vi "Ethernet IP Custom Device Main Page.vi"(8 "error in (no error)":errorcluster, 11 "Node Ptr":T1 format="%.0x") -> (0 "error out":errorcluster)   [LabVIEW 2011, in "Ethernet IP Custom Device Custom Device.lvlib"]
uses:
  Ethernet IP Custom Device Custom Device.lvlib
  <vilib>/NI Veristand/Custom Device API/Custom Device Item Ref.ctl
  <vilib>/NI Veristand/Custom Device API/Custom Device Channel.ctl
  <vilib>/NI Veristand/Custom Device API/Custom Device Channel Type.ctl
  Ethernet IP Global Strings.vi
  <vilib>/NI Veristand/Custom Device API/Get Item Property (I32).vi
  <vilib>/NI Veristand/Custom Device API/Set Item Property (String).vi
  <vilib>/NI Veristand/Custom Device API/Set Item Property (Path).vi
  Ethernet IP Global GUIDs.vi
  <vilib>/NI Veristand/Custom Device API/Set Item Property (I32).vi
  <vilib>/NI Veristand/Custom Device API/Get Item Property (String).vi
  <vilib>/NI Veristand/Custom Device API/Get Item Property (Path).vi
  <vilib>/NI Veristand/Custom Device API/Custom Device API.lvlib
panel:
  in  "Import Selected File":bool
  in  "Path to L5K file":path
  in  "Update Rate (ms)":i32
  in  "Communication Timeout (ms)":i32
  in  "Logix Slot":u16
  in  "Backplane Port":u16
  in  "PLC Address (IP Address)":string
  in  "Header":cluster{"Section Name":string}={"Section Name"="Custom Device Item Settings"}
  in  "Description":string
  in  "Name":string
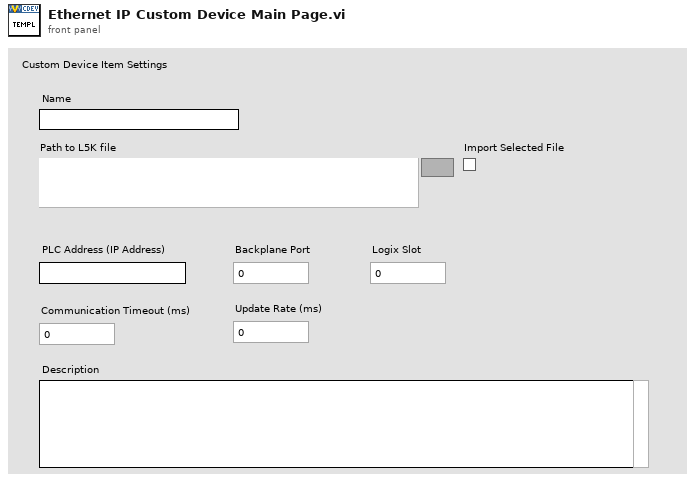
[diagram p1: front panel]
types:
  T1 = typedef "Custom Device API.lvlib/Custom Device Item Ref.ctl" = u64
  T2 = enum8{"Enabled", "Disabled", "Disabled and Grayed Out"}
  T3 = typedef "Custom Device API.lvlib/Custom Device Item Info.ctl" = cluster{"Name":string, "Is Channel":bool, "GUID":string}
  T4 = typedef "Custom Device API.lvlib/Custom Device Channel.ctl" = cluster{"Type":T5, "Units":string, "Default Value":dbl, "Faultable":bool, "Scalable":bool}
  T5 = typedef "Custom Device API.lvlib/Custom Device Channel Type.ctl" = enum16{"Input", "Output"}
  T6 = typedef "Custom Device API.lvlib/Custom Device Commands.ctl" = enum16{"Default", "Item renamed", "Shutdown", "Dynamic button pressed"}
  T7 = typedef "Ethernet IP Custom Device Custom Device.lvlib/L5K Internal Data.ctl" = cluster{"L5K Entire String":string, "L5K Extractred String Array":string[], "IP address from CommPath":string, "Configured Tags":T8[], "Data String Array":string[], "Unconfigured Tags":T8[], "# Tags":i32}
  T8 = typedef "Ethernet IP Custom Device Custom Device.lvlib/L5K Tag.ctl" = cluster{"Tag Name":string, "Data Type":T9, "Data Type String":string, "Array Size":i32, "Description":string, "Input?":bool, "Channel Name":string}
  T9 = typedef "Ethernet IP Custom Device Custom Device.lvlib/L5K Data Types.ctl" = enum16{"SINT", "INT", "DINT", "REAL", "BOOL"}
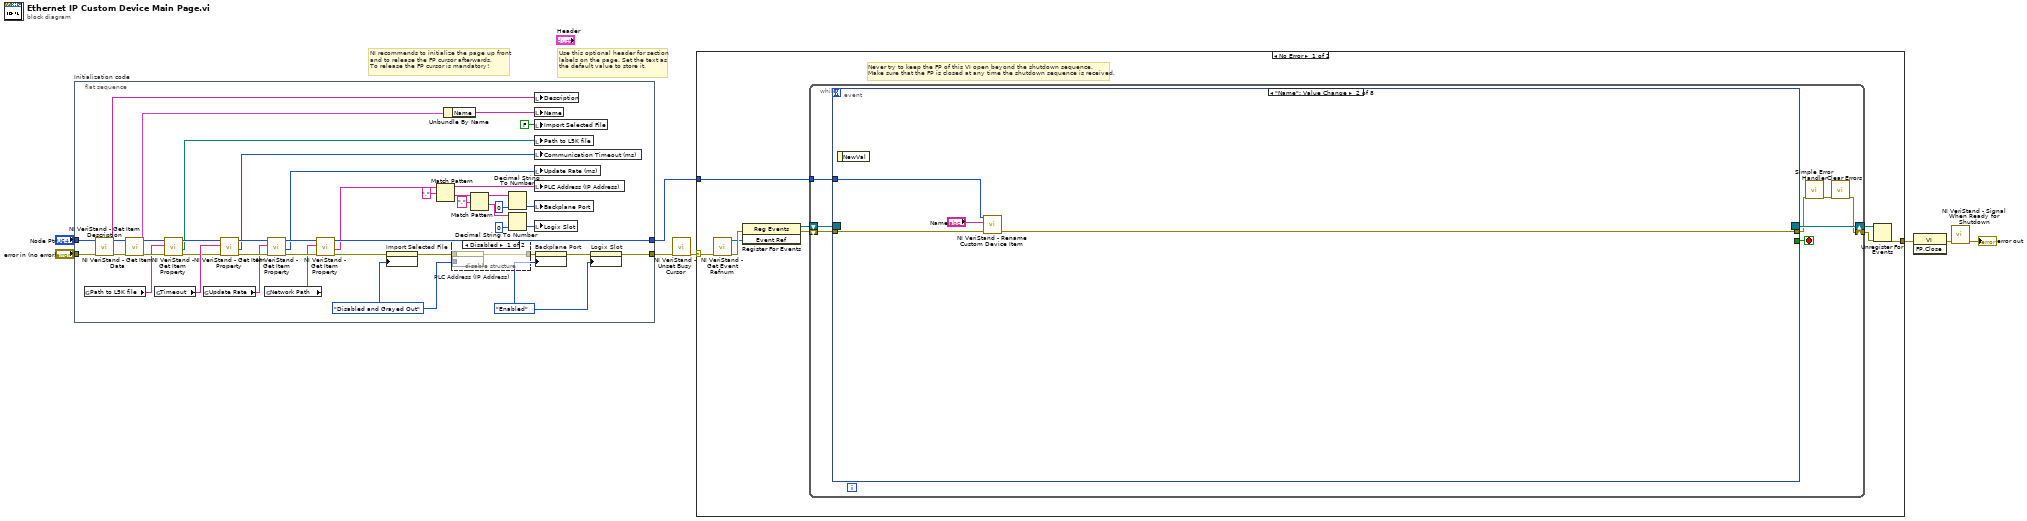
[diagram p0: block diagram]
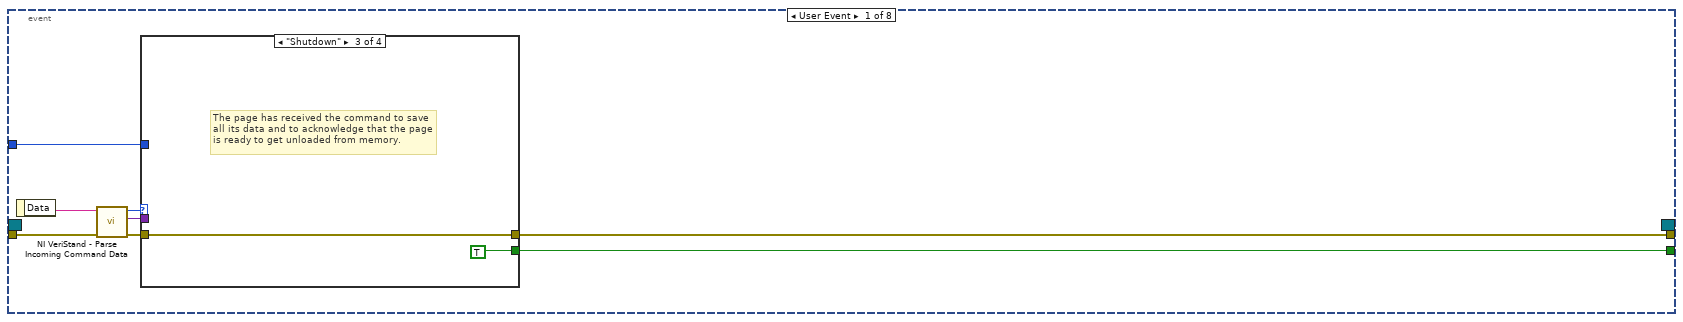
[diagram p2: hidden frame]
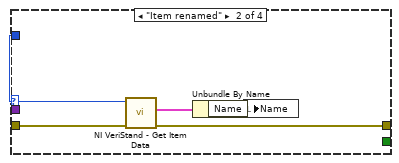
[diagram p4: hidden frame]
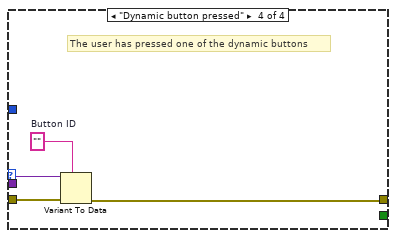
[diagram p5: hidden frame]
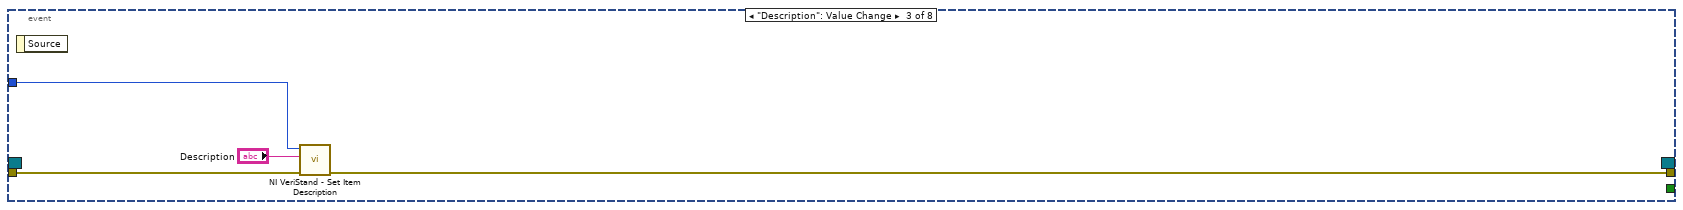
[diagram p6: hidden frame]
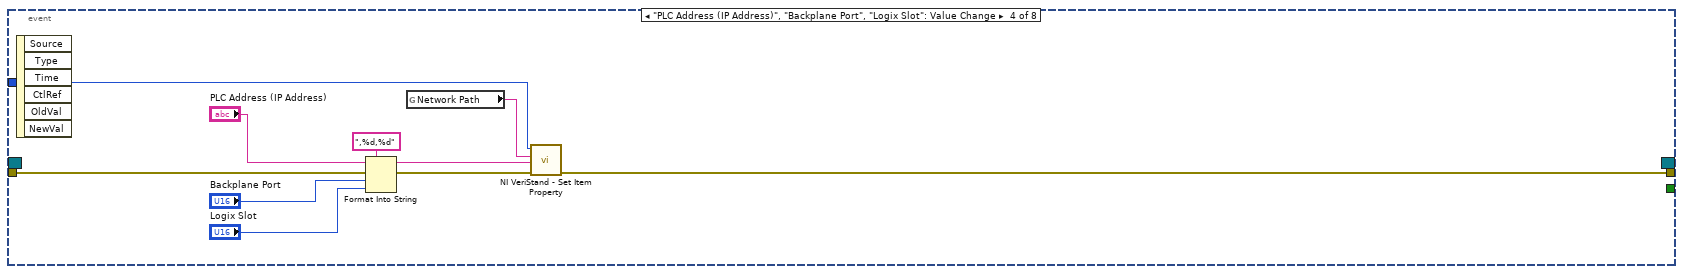
[diagram p7: hidden frame]
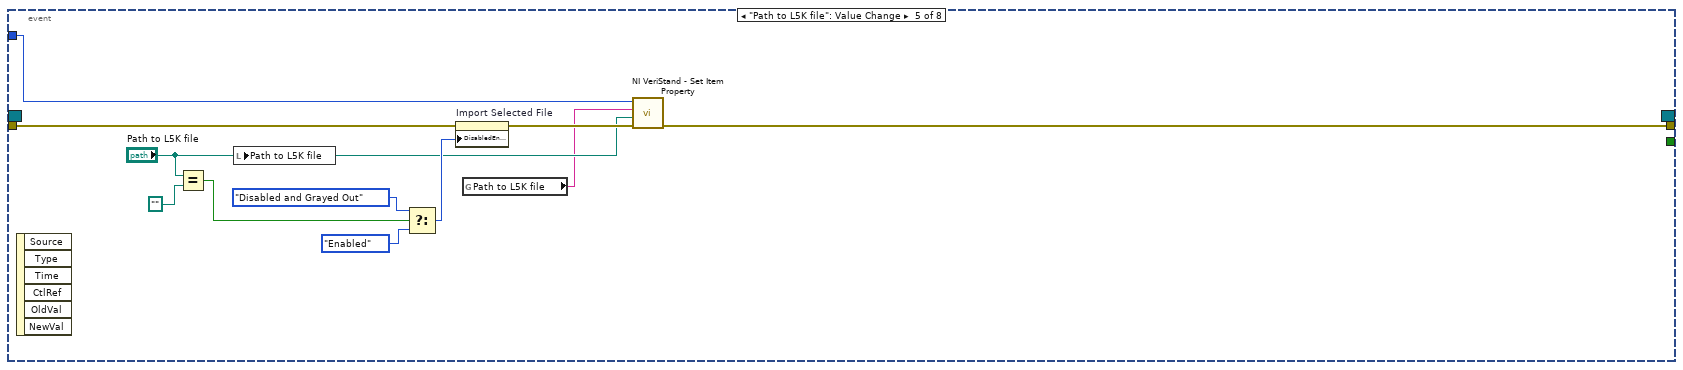
[diagram p8: hidden frame]
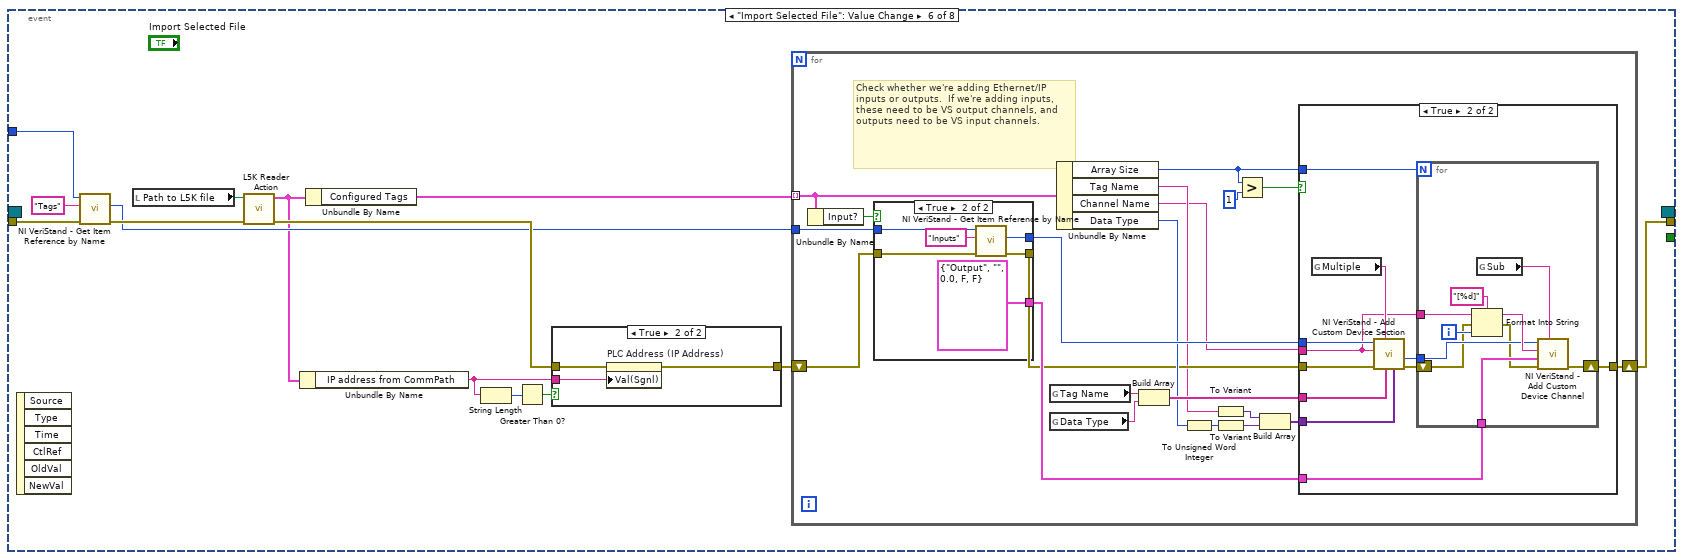
[diagram p9: hidden frame]
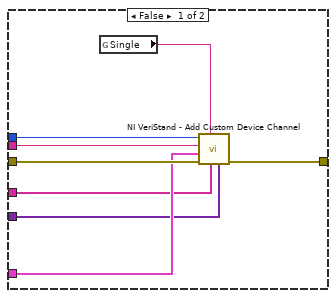
[diagram p10: hidden frame]
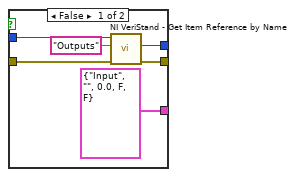
[diagram p11: hidden frame]
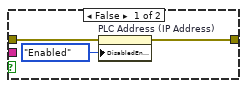
[diagram p12: hidden frame]
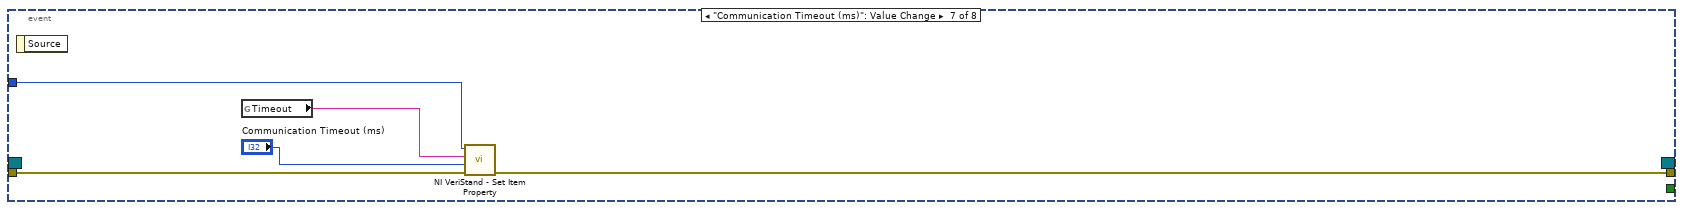
[diagram p13: hidden frame]
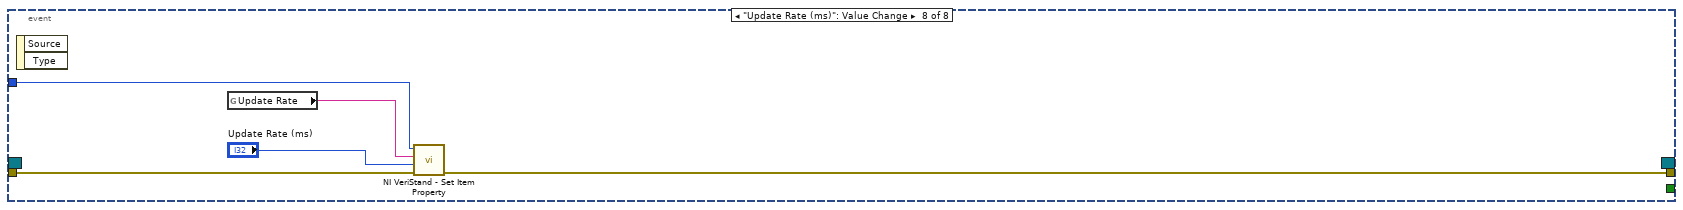
[diagram p14: hidden frame]
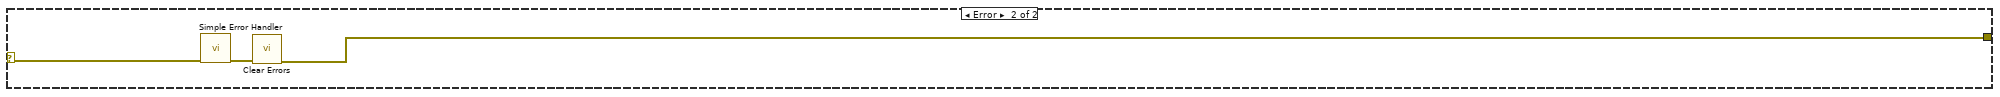
[diagram p15: hidden frame]
diagram:
  # "Use this optional header for section labels on the page. Set the text as the default value to store it."
  # "NI recommends to initialize the page up front\nand to release the FP cursor afterwards.\nTo release the FP cursor is mandatory!"
  n1 = flat-sequence "Initialization code" {
    tunnel: "error in (no error)" -> [w49]
    tunnel: "Node Ptr" -> [w48]
    tunnel: [w20] -> w4
    tunnel: [w27] -> w1
    frame #0 {
      w19 = T2."Enabled" ("Disabled")
      w16 = T2."Disabled and Grayed Out" ("Disabled")
      n2 = global read "Ethernet IP Global Strings.vi" "Path to L5K file"() -> (w10:string)
      n3 = call <vilib>:"NI VeriStand - Get Item Description.vi"("error in (no error)"=w49, "Item Ref in"=w48) -> ("error out"=w46:errorcluster, "Description"=w47:string, "Item Ref out"=w50:T1)  [unwired: 7 out]
      n4 = call <vilib>:"NI VeriStand - Get Item Data.vi"("error in (no error)"=w46, "Item Ref in"=w50) -> ("error out"=w13:errorcluster, "Item Info"=w45:T3, "Item Ref out"=w15:T1)  [unwired: 7 out]
      n5 = global read "Ethernet IP Global Strings.vi" "Timeout"() -> (w33:string)
      n6 = call-poly <vilib>:"NI VeriStand - Get Item Property.vi"("error in (no error)"=w13, "Property Name"=w10, "Item Ref in"=w15) -> ("error out"=w12:errorcluster, "Value"=w9:path, "Item Ref out"=w14:T1)  [unwired: 5 in, 1 out]
      n7 = global read "Ethernet IP Global Strings.vi" "Update Rate"() -> (w32:string)
      n8 = call-poly <vilib>:"NI VeriStand - Get Item Property.vi"("error in (no error)"=w12, "Property Name"=w33, "Item Ref in"=w14) -> ("error out"=w41:errorcluster, "Value"=w30:i32, "Item Ref out"=w43:T1)  [unwired: 5 in, 1 out]
      n9 = global read "Ethernet IP Global Strings.vi" "Network Path"() -> (w31:string)
      n10 = call-poly <vilib>:"NI VeriStand - Get Item Property.vi"("error in (no error)"=w41, "Property Name"=w32, "Item Ref in"=w43) -> ("error out"=w40:errorcluster, "Value"=w28:i32, "Item Ref out"=w42:T1)  [unwired: 5 in, 1 out]
      n11 = call-poly <vilib>:"NI VeriStand - Get Item Property.vi"("error in (no error)"=w40, "Property Name"=w31, "Item Ref in"=w42) -> ("error out"=w18:errorcluster, "Value"=w24:string, "Item Ref out"=w27:T1)  [unwired: 5 in, 1 out]
      n12 = property on="Import Selected File" class="Bool (strict)"(error in=w18, "DisabledEnum"=w16) -> (error out=w17:errorcluster)  [unwired: 1 in, 1 out]
      n13 = Match Pattern(string=w24, regular expression=",") -> (before substring=w25:string, after substring=w23:string)  [unwired: 1 in, 2 out]
      n14 = Unbundle By Name(w45) -> ("Name"=w44:string)
      n15 = disable-structure shown="Disabled" {
        disable-tunnel: [w53 w54] -> w22
        disable-tunnel: w17 -> [w52 w54]
        disable-tunnel: w16 -> [w51 _]
        frame Disabled {
          n16 = property on="PLC Address (IP Address)" class="Str"(error in=w52, "DisabledEnum"=w51) -> (error out=w53:errorcluster)  [unwired: 1 in, 1 out]
        }
        frame Enabled {
        }
      }
      n17 = Match Pattern(string=w23, regular expression=",") -> (before substring=w37:string, after substring=w36:string)  [unwired: 1 in, 2 out]
      n18 = Decimal String To Number(string=w37, default (0L)=u16 0 ("default (0 I32)")) -> (number=w34:u16)  [unwired: 1 in, 1 out]
      n19 = Decimal String To Number(string=w36, default (0L)=u16 0 ("default (0 I32)")) -> (number=w29:u16)  [unwired: 1 in, 1 out]
      n20 = local write "Description"(w47) -> ()
      n21 = local write "Name"(w44) -> ()
      n22 = local write "Import Selected File"(FALSE ("Import Selected File")) -> ()
      n23 = local write "Path to L5K file"(w9) -> ()
      n24 = local write "Communication Timeout (ms)"(w30) -> ()
      n25 = local write "Update Rate (ms)"(w28) -> ()
      n26 = local write "PLC Address (IP Address)"(w25) -> ()
      n27 = local write "Backplane Port"(w34) -> ()
      n28 = local write "Logix Slot"(w29) -> ()
      n29 = property on="Backplane Port" class="DigNum (strict)"(error in=w22, "DisabledEnum"=w19) -> (error out=w21:errorcluster)  [unwired: 1 in, 1 out]
      n30 = property on="Logix Slot" class="DigNum (strict)"(error in=w21, "DisabledEnum"=w19) -> (error out=w20:errorcluster)  [unwired: 1 in, 1 out]
    }
  }
  n31 = call <vilib>:"NI VeriStand - Unset Busy Cursor.vi"("error in (no error)"=w4) -> ("error out"=w3:errorcluster)  [unwired: 10 out]
  n32 = case shown="No Error" w3 {
    selector: w3 -> [w55 w215]
    tunnel: [w60 w213] -> w8
    tunnel: w1 -> [w56 _]
    frame No Error {
      # "Never try to keep the FP of this VI open beyond the shutdown sequence.\nMake sure that the FP is closed at any time the shutdown sequence is received."
      n33 = call <vilib>:"NI VeriStand - Get Event Refnum.vi"("error in (no error)"=w55) -> ("error out"=w63:errorcluster, "Event Ref"=w59:refnum<user-event>)  [unwired: 9 out]
      n34 = register-events(error in=w63, w59) -> (reference out=w57:refnum<event-registration>, error out=w58:errorcluster)  [unwired: 1 in]
      n35 = while {
        tunnel: w56 -> [w67]
        shift-right: [w64] -> w61
        shift-left: w58 -> [w70]
        shift-right: [w71] -> w62
        shift-left: w57 -> [w69]
        stop <- w68 stop-if-true
        n36 = event shown="[1] \"Name\": Value Change" {
          selector: w69 -> [_ _ _ _ _ _ _ _]
          dyn-events: [_ _ _ _ _ _ _ _] -> w71
          timeout: _ -> [_ _ _ _ _ _ _ _]
          tunnel: w70 -> [w79 w95 w98 w105 w115 w126 w204 w210]
          tunnel: [w75 _ _ _ _ _ _ _] -> w68
          tunnel: [w74 w94 w97 w109 w113 w128 w207 w212] -> w66
          tunnel: w67 -> [w73 w93 w99 w108 w112 w127 w206 w211]
          event User Event {
            n37 = event-data() -> ("Data"=w78:string)  [unwired: 1 out]
            n38 = call <vilib>:"NI VeriStand - Parse Incoming Command Data.vi"("error in (no error)"=w79, "Incoming data"=w78) -> ("error out"=w77:errorcluster, "Outgoing data"=w72:variant, "Action"=w76:T6)  [unwired: 7 out]
            n39 = case shown="\"Shutdown\"" w76 {
              tunnel: w77 -> [w80 w85 w86 w91]
              tunnel: [_ _ TRUE _] -> w75
              tunnel: [w80 w82 w86 w88] -> w74
              tunnel: w73 -> [_ w84 _ _]
              tunnel: w72 -> [_ _ _ w90]
              frame "Default", Default {
              }
              frame "Item renamed" {
                n40 = call <vilib>:"NI VeriStand - Get Item Data.vi"("error in (no error)"=w85, "Item Ref in"=w84) -> ("error out"=w82:errorcluster, "Item Info"=w83:T3)  [unwired: 8 out]
                n41 = Unbundle By Name(w83) -> ("Name"=w81:string)
                n42 = local write "Name"(w81) -> ()
              }
              frame "Shutdown" {
                # "The page has received the command to save all its data and to acknowledge that the page is ready to get unloaded from memory."
              }
              frame "Dynamic button pressed" {
                w89 = ""  # Button ID
                # "The user has pressed one of the dynamic buttons"
                n43 = Variant To Data(error in=w91, type=w89, Variant=w90) -> (error out=w88:errorcluster)  [unwired: 1 out]
              }
            }
          }
          event "Name": Value Change {
            n44 = event-data() -> ()  [unwired: 2 out]
            n45 = call <vilib>:"NI VeriStand - Rename Custom Device Item.vi"("error in (no error)"=w95, "New Name"="Name", "Item Ref in"=w93) -> ("error out"=w94:errorcluster)  [unwired: 8 out]
          }
          event "Description": Value Change {
            n46 = event-data() -> ()  [unwired: 2 out]
            n47 = call <vilib>:"NI VeriStand - Set Item Description.vi"("error in (no error)"=w98, "Description"="Description", "Item Ref in"=w99) -> ("error out"=w97:errorcluster)  [unwired: 8 out]
          }
          event "PLC Address (IP Address)", "Backplane Port", "Logix Slot": Value Change {
            n48 = event-data() -> ()  [unwired: 7 out]
            n49 = Format Into String(format string=",%d,%d", initial string="PLC Address (IP Address)", error in=w105, "Backplane Port", "Logix Slot") -> (resulting string=w103:string, error out=w104:errorcluster)
            n50 = global read "Ethernet IP Global Strings.vi" "Network Path"() -> (w107:string)
            n51 = call-poly <vilib>:"NI VeriStand - Set Item Property.vi"("error in (no error)"=w104, "Value"=w103, "Property Name"=w107, "Item Ref in"=w108) -> ("error out"=w109:errorcluster)  [unwired: 5 in, 2 out]
          }
          event "Path to L5K file": Value Change {
            n52 = event-data() -> ()  [unwired: 7 out]
            n53 = Equal?(x="Path to L5K file", y=path "") -> (x = y?=w119:bool)
            n54 = local write "Path to L5K file"("Path to L5K file") -> ()
            n55 = Select(t=T2."Disabled and Grayed Out" ("Disabled"), s=w119, f=T2."Enabled" ("Disabled")) -> (s? t:f=w116:T2)
            n56 = property on="Import Selected File" class="Bool (strict)"(error in=w115, "DisabledEnum"=w116) -> (error out=w114:errorcluster)  [unwired: 1 in, 1 out]
            n57 = global read "Ethernet IP Global Strings.vi" "Path to L5K file"() -> (w110:string)
            n58 = call-poly <vilib>:"NI VeriStand - Set Item Property.vi"("error in (no error)"=w114, "Value"="Path to L5K file", "Property Name"=w110, "Item Ref in"=w112) -> ("error out"=w113:errorcluster)  [unwired: 5 in, 2 out]
          }
          event "Import Selected File": Value Change {
            n59 = event-data() -> ()  [unwired: 7 out]
            n60 = call <vilib>:"NI VeriStand - Get Item Reference by Name.vi"("error in (no error)"=w126, "Item Name"="Tags", "Parent Ref in"=w127) -> ("error out"=w124:errorcluster, "Item Ref"=w123:T1)  [unwired: 5 in, 2 out]
            n61 = local read "Path to L5K file"() -> (w121:path)
            n62 = call "L5K Reader Action.vi"("error in"=w124, "L5K File Path"=w121) -> ("error out"=w131:errorcluster, "L5K Information"=w122:T7)  [unwired: 7 in, 1 out]
            n63 = Unbundle By Name(w122) -> ("IP address from CommPath"=w132:string)
            n64 = Unbundle By Name(w122) -> ("Configured Tags"=w130:T8[])
            n65 = String Length(string=w132) -> (length=w134:i32)
            n66 = Greater Than 0?(x=w134) -> (x > 0?=w133:bool)
            n67 = case shown="True" w133 {
              tunnel: w132 -> [_ w202]
              tunnel: w131 -> [w198 w201]
              tunnel: [w197 w200] -> w129
              frame False {
                n68 = property on="PLC Address (IP Address)" class="Str"(error in=w198, "DisabledEnum"=T2."Enabled" ("Disabled")) -> (error out=w197:errorcluster)  [unwired: 1 in, 1 out]
              }
              frame True {
                n69 = property on="PLC Address (IP Address)" class="Str"(error in=w201, "Val(Sgnl)"=w202) -> (error out=w200:errorcluster)  [unwired: 1 in, 1 out]
              }
            }
            n70 = for {
              tunnel: w123 -> [w145]
              shift-right: [w143] -> w128
              shift-left: w129 -> [w138]
              tunnel: w130 -> [w139] mode=indexing
              # "Check whether we're adding Ethernet/IP\ninputs or outputs.  If we're adding inputs,\nthese need to be VS output channels, and\noutputs need to be VS input channels."
              n71 = Unbundle By Name(w139) -> ("Input?"=w142:bool)
              n72 = case shown="True" w142 {
                tunnel: [T4 {"Type"=enum."Input", "Units"="", "Default Value"=0.0, "Faultable"=FALSE, "Scalable"=FALSE} ("Channel") T4 {"Type"=enum."Output", "Units"="", "Default Value"=0.0, "Faultable"=FALSE, "Scalable"=FALSE} ("Channel")] -> w155
                tunnel: w145 -> [w189 w195]
                tunnel: [w187 w194] -> w144
                tunnel: w138 -> [w186 w192]
                tunnel: [w185 w191] -> w137
                frame False {
                  n73 = call <vilib>:"NI VeriStand - Get Item Reference by Name.vi"("error in (no error)"=w186, "Item Name"="Outputs", "Parent Ref in"=w189) -> ("error out"=w185:errorcluster, "Item Ref"=w187:T1)  [unwired: 5 in, 2 out]
                }
                frame True {
                  n74 = call <vilib>:"NI VeriStand - Get Item Reference by Name.vi"("error in (no error)"=w192, "Item Name"="Inputs", "Parent Ref in"=w195) -> ("error out"=w191:errorcluster, "Item Ref"=w194:T1)  [unwired: 5 in, 2 out]
                }
              }
              n75 = global read "Ethernet IP Global Strings.vi" "Tag Name"() -> (w147:string)
              n76 = global read "Ethernet IP Global Strings.vi" "Data Type"() -> (w146:string)
              n77 = Unbundle By Name(w139) -> ("Array Size"=w140:i32, "Tag Name"=w136:string, "Channel Name"=w135:string, "Data Type"=w141:T9)
              n78 = Build Array(w147, w146) -> (w150:string[])
              n79 = To Unsigned Word Integer(number=w141) -> (unsigned 16bit integer=w149:u16)
              n80 = To Variant(anything=w136) -> (Variant=w148:variant)
              n81 = To Variant(anything=w149) -> (Variant=w152:variant)
              n82 = Greater?(x=w140, y=1) -> (0:w153:bool)
              n83 = Build Array(w148, w152) -> (w151:variant[])
              n84 = case shown="True" w153 {
                tunnel: w137 -> [w163 w172]
                tunnel: w155 -> [w162 w164]
                tunnel: w135 -> [w156 w166]
                tunnel: w151 -> [w160 w174]
                tunnel: w150 -> [w161 w173]
                tunnel: w144 -> [w159 w169]
                tunnel: [w157 w167] -> w143
                tunnel: w140 -> [_ w165]
                frame False {
                  n85 = global read "Ethernet IP Global GUIDs.vi" "Single"() -> (w158:string)
                  n86 = call <vilib>:"NI VeriStand - Add Custom Device Channel.vi"("Property Values"=w160, "Property names"=w161, "GUID (Default Channel)"=w158, "error in (no error)"=w163, "Channel"=w162, "Channel Name"=w156, "Parent Ref in"=w159) -> ("error out"=w157:errorcluster)  [unwired: 1 in, 3 out]
                }
                frame True {
                  n87 = global read "Ethernet IP Global GUIDs.vi" "Multiple"() -> (w168:string)
                  n88 = call <vilib>:"NI VeriStand - Add Custom Device Section.vi"("Property Values"=w174, "Property names"=w173, "GUID (Default Section)"=w168, "error in (no error)"=w172, "Section Name"=w166, "Parent Ref in"=w169) -> ("error out"=w170:errorcluster, "Section Ptr"=w171:T1)  [unwired: 2 in, 2 out]
                  n89 = for {
                    N: w165 -> [_]
                    tunnel: w171 -> [w181]
                    tunnel: w164 -> [w180]
                    shift-right: [w178] -> w167
                    shift-left: w170 -> [w176]
                    tunnel: w166 -> [w177]
                    i -> [w184]
                    n90 = Format Into String(format string="[%d]", initial string=w177, error in=w176, w184) -> (resulting string=w182:string, error out=w175:errorcluster)
                    n91 = global read "Ethernet IP Global GUIDs.vi" "Sub"() -> (w179:string)
                    n92 = call <vilib>:"NI VeriStand - Add Custom Device Channel.vi"("GUID (Default Channel)"=w179, "error in (no error)"=w175, "Channel"=w180, "Channel Name"=w182, "Parent Ref in"=w181) -> ("error out"=w178:errorcluster)  [unwired: 3 in, 3 out]
                  }
                }
              }
            }
          }
          event "Communication Timeout (ms)": Value Change {
            n93 = event-data() -> ()  [unwired: 2 out]
            n94 = global read "Ethernet IP Global Strings.vi" "Timeout"() -> (w205:string)
            n95 = call-poly <vilib>:"NI VeriStand - Set Item Property.vi"("error in (no error)"=w204, "Value"="Communication Timeout (ms)", "Property Name"=w205, "Item Ref in"=w206) -> ("error out"=w207:errorcluster)  [unwired: 5 in, 2 out]
          }
          event "Update Rate (ms)": Value Change {
            n96 = event-data() -> ()  [unwired: 3 out]
            n97 = global read "Ethernet IP Global Strings.vi" "Update Rate"() -> (w209:string)
            n98 = call-poly <vilib>:"NI VeriStand - Set Item Property.vi"("error in (no error)"=w210, "Value"="Update Rate (ms)", "Property Name"=w209, "Item Ref in"=w211) -> ("error out"=w212:errorcluster)  [unwired: 5 in, 2 out]
          }
        }
        n99 = call <vilib>:"Simple Error Handler.vi"("error in (no error)"=w66) -> ("error out"=w65:errorcluster)  [unwired: 1 in, 7 out]
        n100 = call <vilib>:"Clear Errors.vi"("error in (no error)"=w65) -> ("error out"=w64:errorcluster)  [unwired: 6 out]
      }
      n101 = Unregister For Events(event registration refnum=w62, error in=w61) -> (error out=w60:errorcluster)
    }
    frame Error {
      n102 = call <vilib>:"Simple Error Handler.vi"("error in (no error)"=w215) -> ("error out"=w214:errorcluster)  [unwired: 1 in, 7 out]
      n103 = call <vilib>:"Clear Errors.vi"("error in (no error)"=w214) -> ("error out"=w213:errorcluster)  [unwired: 6 out]
    }
  }
  n104 = invoke class="VI" method="FP.Close"(error in=w8) -> (error out=w7:errorcluster)  [unwired: 2 in, 2 out]
  n105 = call <vilib>:"NI VeriStand - Signal When Ready for Shutdown.vi"("error in (no error)"=w7) -> ("error out"=→"error out":errorcluster)  [unwired: 10 out]
